vi "Analysis.Data Dump, Result Header to to 1D Str.vi"(10 "Result Summary":T1, 11 "Data List In":string[](array[string])) -> (3 "Data List out":string[](array[string]), 5 "Genealogy Headings":string[](array[string]))   [LabVIEW 2024]
uses:
  Analysis.Result Summary.ctl
  Time/Time.Format Selector.ctl
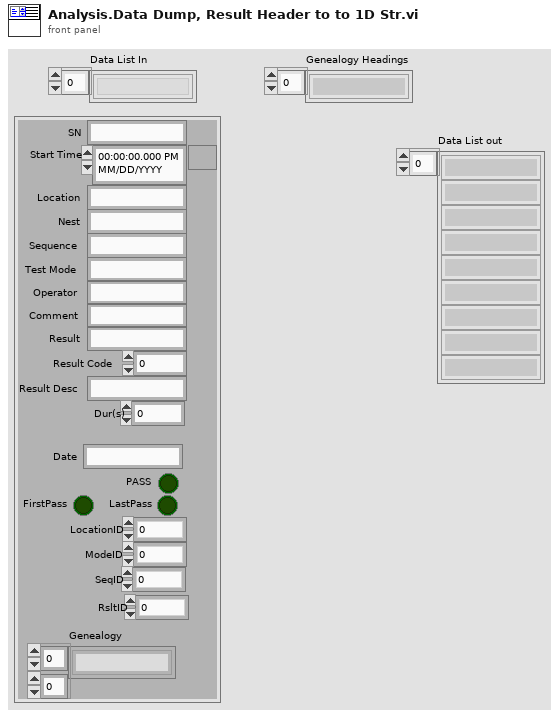
[diagram p1: front panel]
types:
  T1 = typedef "Analysis.Result Summary.ctl" = cluster{"SN":string, "Start Time":timestamp, "Location":string, "Nest":string, "Sequence":string, "Operator":string, "Test Mode":string, "Comment":string, "Result":string, "Result Code":i32, "Result Desc":string, "Date":string, "Dur(s)":dbl, "PASS":bool, "FirstPass":bool, "LastPass":bool, "LocationID":i32, "ModeID":i32, "SeqID":i32, "RsltID":i32, "Genealogy":string[][]}
  T2 = typedef "Time.Format Selector.ctl" = enum16{"yyyy/mm/dd HH:MM:S.sss", "yyyy/mm/dd HH:MM:SS", "yyyy-MM-ddTHH:mm:ss[.mmm]", "YYYYMMDD_HHMMSS"}
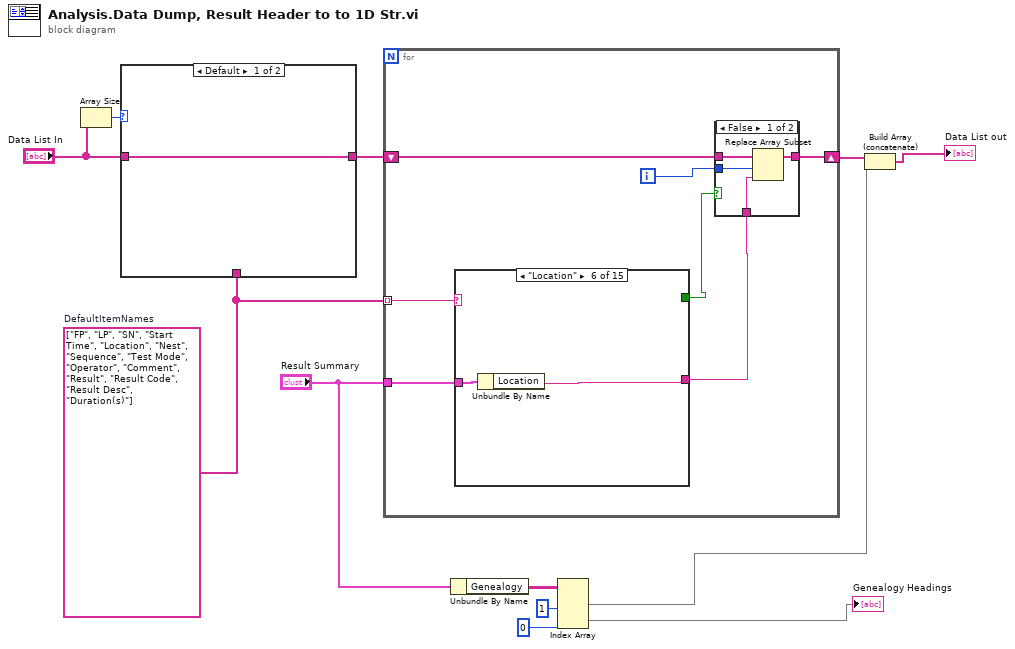
[diagram p0: block diagram]
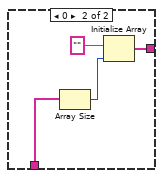
[diagram p2: hidden frame]
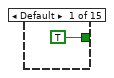
[diagram p4: hidden frame]
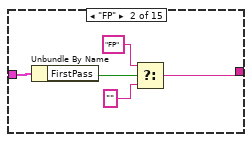
[diagram p5: hidden frame]
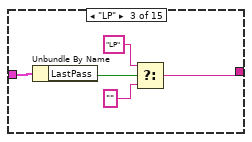
[diagram p6: hidden frame]
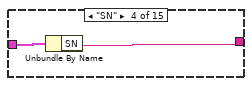
[diagram p7: hidden frame]
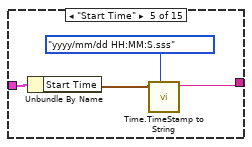
[diagram p8: hidden frame]
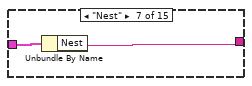
[diagram p9: hidden frame]
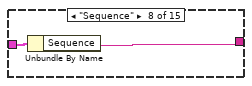
[diagram p10: hidden frame]
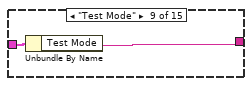
[diagram p11: hidden frame]
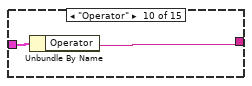
[diagram p12: hidden frame]
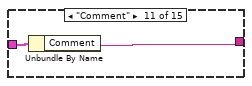
[diagram p13: hidden frame]
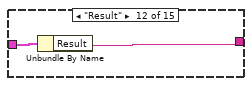
[diagram p14: hidden frame]
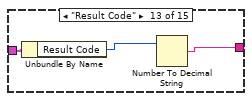
[diagram p15: hidden frame]
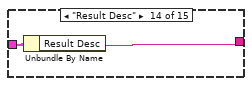
[diagram p16: hidden frame]
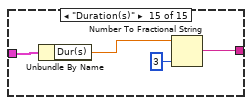
[diagram p17: hidden frame]
diagram:
  w9 = string[] ["FP", "LP", "SN", "Start Time", "Location", "Nest", "Sequence", "Test Mode", "Operator", "Comment", "Result", "Result Code", "Result Desc", "Duration(s)"]  # DefaultItemNames
  n1 = Array Size(array="Data List In") -> (size(s)=w12:i32)
  n2 = case shown="Default" w12 {
    tunnel: [w13 w16] -> w11
    tunnel: "Data List In" -> [w13 _]
    tunnel: w9 -> [_ w15]
    frame Default {
    }
    frame 0 {
      n3 = Array Size(array=w15) -> (size(s)=w14:i32)
      n4 = Initialize Array("", w14) -> (w16:string[])
    }
  }
  n5 = for {
    shift-right: [w23] -> w4
    shift-left: w11 -> [w24]
    tunnel: "Result Summary" -> [w21]
    tunnel: w9 -> [w20] mode=indexing
    i -> [w19]
    n6 = case shown="\"Location\"" w20 {
      tunnel: [_ w33 w38 w41 w44 w47 w49 w51 w53 w55 w57 w59 w61 w64 w66] -> w22
      tunnel: w21 -> [_ w35 w40 w42 w46 w48 w50 w52 w54 w56 w58 w60 w63 w65 w69]
      tunnel: [TRUE _ _ _ _ _ _ _ _ _ _ _ _ _ _] -> w18
      frame Default {
      }
      frame "FP" {
        n7 = Unbundle By Name(w35) -> ("FirstPass"=w34:bool)
        n8 = Select(t="FP", s=w34, f="") -> (s? t:f=w33:string)
      }
      frame "LP" {
        n9 = Unbundle By Name(w40) -> ("LastPass"=w39:bool)
        n10 = Select(t="LP", s=w39, f="") -> (s? t:f=w38:string)
      }
      frame "SN" {
        n11 = Unbundle By Name(w42) -> ("SN"=w41:string)
      }
      frame "Start Time" {
        n12 = Unbundle By Name(w46) -> ("Start Time"=w45:timestamp)
        n13 = call "Time.TimeStamp to String.vi"("TimeFormat"=Time.Format_Selector."yyyy/mm/dd HH:MM:S.sss", "Time Stamp in"=w45) -> ("Time String Out"=w44:string)  [unwired: 9 in]
      }
      frame "Location" {
        n14 = Unbundle By Name(w48) -> ("Location"=w47:string)
      }
      frame "Nest" {
        n15 = Unbundle By Name(w50) -> ("Nest"=w49:string)
      }
      frame "Sequence" {
        n16 = Unbundle By Name(w52) -> ("Sequence"=w51:string)
      }
      frame "Test Mode" {
        n17 = Unbundle By Name(w54) -> ("Test Mode"=w53:string)
      }
      frame "Operator" {
        n18 = Unbundle By Name(w56) -> ("Operator"=w55:string)
      }
      frame "Comment" {
        n19 = Unbundle By Name(w58) -> ("Comment"=w57:string)
      }
      frame "Result" {
        n20 = Unbundle By Name(w60) -> ("Result"=w59:string)
      }
      frame "Result Code" {
        n21 = Unbundle By Name(w63) -> ("Result Code"=w62:i32)
        n22 = Number To Decimal String(number=w62) -> (decimal integer string=w61:string)  [unwired: 1 in]
      }
      frame "Result Desc" {
        n23 = Unbundle By Name(w65) -> ("Result Desc"=w64:string)
      }
      frame "Duration(s)" {
        n24 = Unbundle By Name(w69) -> ("Dur(s)"=w68:dbl)
        n25 = Number To Fractional String(number=w68, precision (6)=i16 3) -> (F-format string=w66:string)  [unwired: 2 in]
      }
    }
    n26 = case shown="False" w18 {
      tunnel: w24 -> [w28 w29]
      tunnel: [w27 w29] -> w23
      tunnel: w22 -> [w26 _]
      tunnel: w19 -> [w25 _]
      frame False {
        n27 = Replace Array Subset(array=w28, new element=w26, index=w25) -> (w27:string[])
      }
      frame True {
      }
    }
  }
  n28 = Unbundle By Name("Result Summary") -> ("Genealogy"=w7:string[][])
  n29 = Index Array(array=w7, index (col) #1=1 ("disabled index (col)"), index (col) #2=0 ("disabled index (col)")) -> (element #1=w2:string[], element #2=→"Genealogy Headings":string[])  [unwired: 2 in]
  n30 = Build Array (concatenate)(w4, w2) -> (→"Data List out":string[])
